vi "Transform Vector To Screen Space.vi"() -> ()   [LabVIEW 2020, in "3D.lvlib"]
uses:
  Vector 3D.ctl
  3D.lvlib
panel:
  in  "a":dbl
  in  "Vector 3D":T1
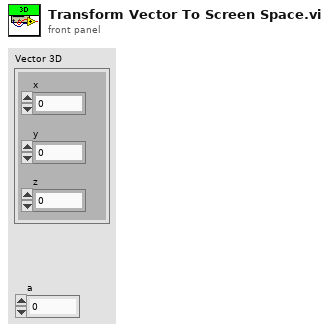
[diagram p1: front panel]
types:
  T1 = typedef "3D.lvlib/Vector 3D.ctl" = cluster{"x":sgl, "y":sgl, "z":sgl}
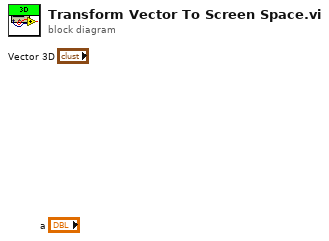
[diagram p0: block diagram]
diagram:
